vi "Update Value by Index.vi"(4 "Raw":dbl, 6 "Timestamp (Now)":dbl, 8 "error in (no error)":errorcluster, 9 "Scaled":dbl, 10 "Index":i32, 11 "Group in":refnum<class "Group.lvclass">) -> (0 "error out":errorcluster, 3 "Group out":refnum<class "Group.lvclass">)   [LabVIEW 2020, in "Vecto.lvlib" / "Group.lvclass"]
uses:
  Group.lvclass
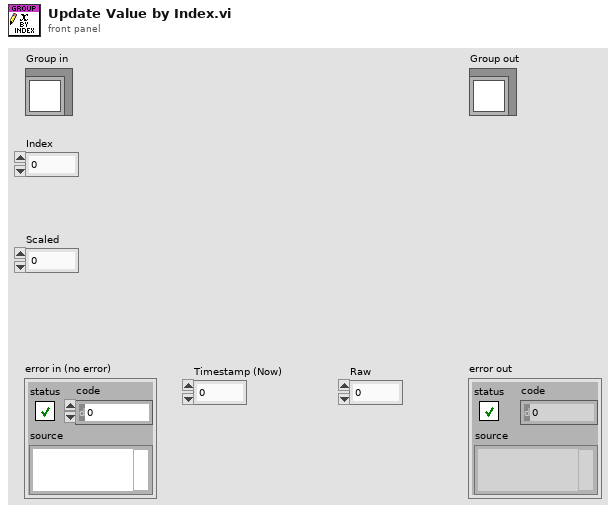
[diagram p1: front panel]
types:
  T1 = typedef "Vecto.lvlib/Group.lvclass/Ref.ctl" = cluster{"Channel Index Map":map{string, i32}, "Channel Info":T2[], "Scaled":dbl[], "Timestamp":dbl[], "Raw":dbl[]}
  T2 = typedef "Vecto.lvlib/Channel Info.ctl" = cluster{"Name":string, "Group":string, "Owning Node":string, "Owning Task":string, "Resource":string}
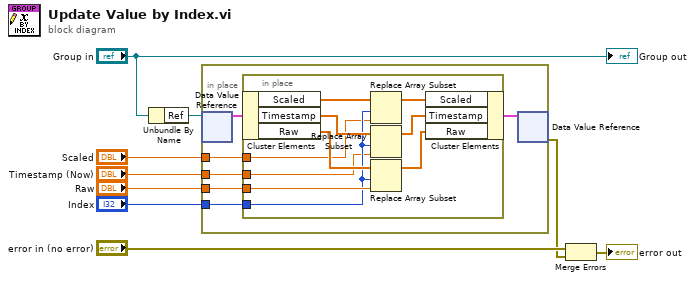
[diagram p0: block diagram]
diagram:
  n1 = Unbundle By Name("Group in") -> ("Ref"=w7:refnum<data-value>)
  n2 = in-place {
    in-place-border: "Scaled" -> [w14]
    in-place-border: "Timestamp (Now)" -> [w13]
    in-place-border: "Raw" -> [w12]
    in-place-border: "Index" -> [w11]
    n3 = in-place-dvr #1(w7) -> (w15:T1)  [unwired: 1 out]
    n4 = in-place {
      in-place-border: w14 -> [w19]
      in-place-border: w13 -> [w20]
      in-place-border: w12 -> [w23]
      in-place-border: w11 -> [w21]
      n5 = in-place-cluster #2(w15) -> ("Scaled"=w25:dbl[], "Timestamp"=w22:dbl[], "Raw"=w24:dbl[])
      n6 = Replace Array Subset(array=w25, new element=w19, index=w21) -> (w18:dbl[])
      n7 = Replace Array Subset(array=w22, new element=w20, index=w21) -> (w17:dbl[])
      n8 = Replace Array Subset(array=w24, new element=w23, index=w21) -> (w16:dbl[])
      n9 = in-place-cluster #2("Scaled"=w18, "Timestamp"=w17, "Raw"=w16) -> (w10:T1)
    }
    n10 = in-place-dvr #1(w10) -> (w1:errorcluster)  [unwired: 1 out]
  }
  n11 = Merge Errors("error in (no error)", w1) -> (→"error out":errorcluster)
  "Group out" <- "Group in"
